vi "DrivePath.vi"(3 "Reinit":bool) -> (0 "Path Follower Error":errorcluster, 1 "Increment":bool)   [LabVIEW 2019]
doc: "A pure-pursuit path-following algorithm configured for a swerve drive. Feed-forward and feed-back controllers are combined to produce unitless drive commands. This VI is designed to integrated with the FRC 4265 Autonomous Path Planner. The Search Window can be specified in seconds - longer search windows are more robust to recovering from large deviations from the path but may cause the robot to \"jump\" ahead when following tight loops or turns. The Look-Ahead Time specifies the furthest ahead the pursuit point can be.\n\nParameters:\n1. acceptable distance error --> (in) [0,614.25]\n2. acceptable angle error --> (deg) [0,180]\n3. path follow timeout --> (ms) [0,15000] set to -1 for no timeout\n3. name of the autonomous path\n4. specifiy whether or not the robot can add a suffix to the selected path name {normal,robot_suffix}"
uses:
  sensors.vi
  dsinstructions.vi
  autoninfo.vi
panel:
  in  "Dist Kd":dbl
  in  "Turn Kd":dbl
  in  "Turn Ki":dbl
  in  "Turn Kp":dbl
  in  "Dist Ki":dbl
  in  "Dist Kp":dbl
  in  "file_name":string
  in  "timeout":dbl
  in  "acceptable angle error":dbl
  in  "acceptable distance error":dbl
  out "PID Strafe":cluster{"Goal Wheel Position":dbl, dbl}(graph)
  out "PID Heading":cluster{"Goal Wheel Position":dbl, dbl}(graph)
  out "Path and Robot Pose":cluster{dbl[], dbl[]}[](graph)
  in  "Plot":bool
  in  "Max Look-Ahead Time (s)":dbl=0.5
  in  "Search Window (s)":dbl=2.0
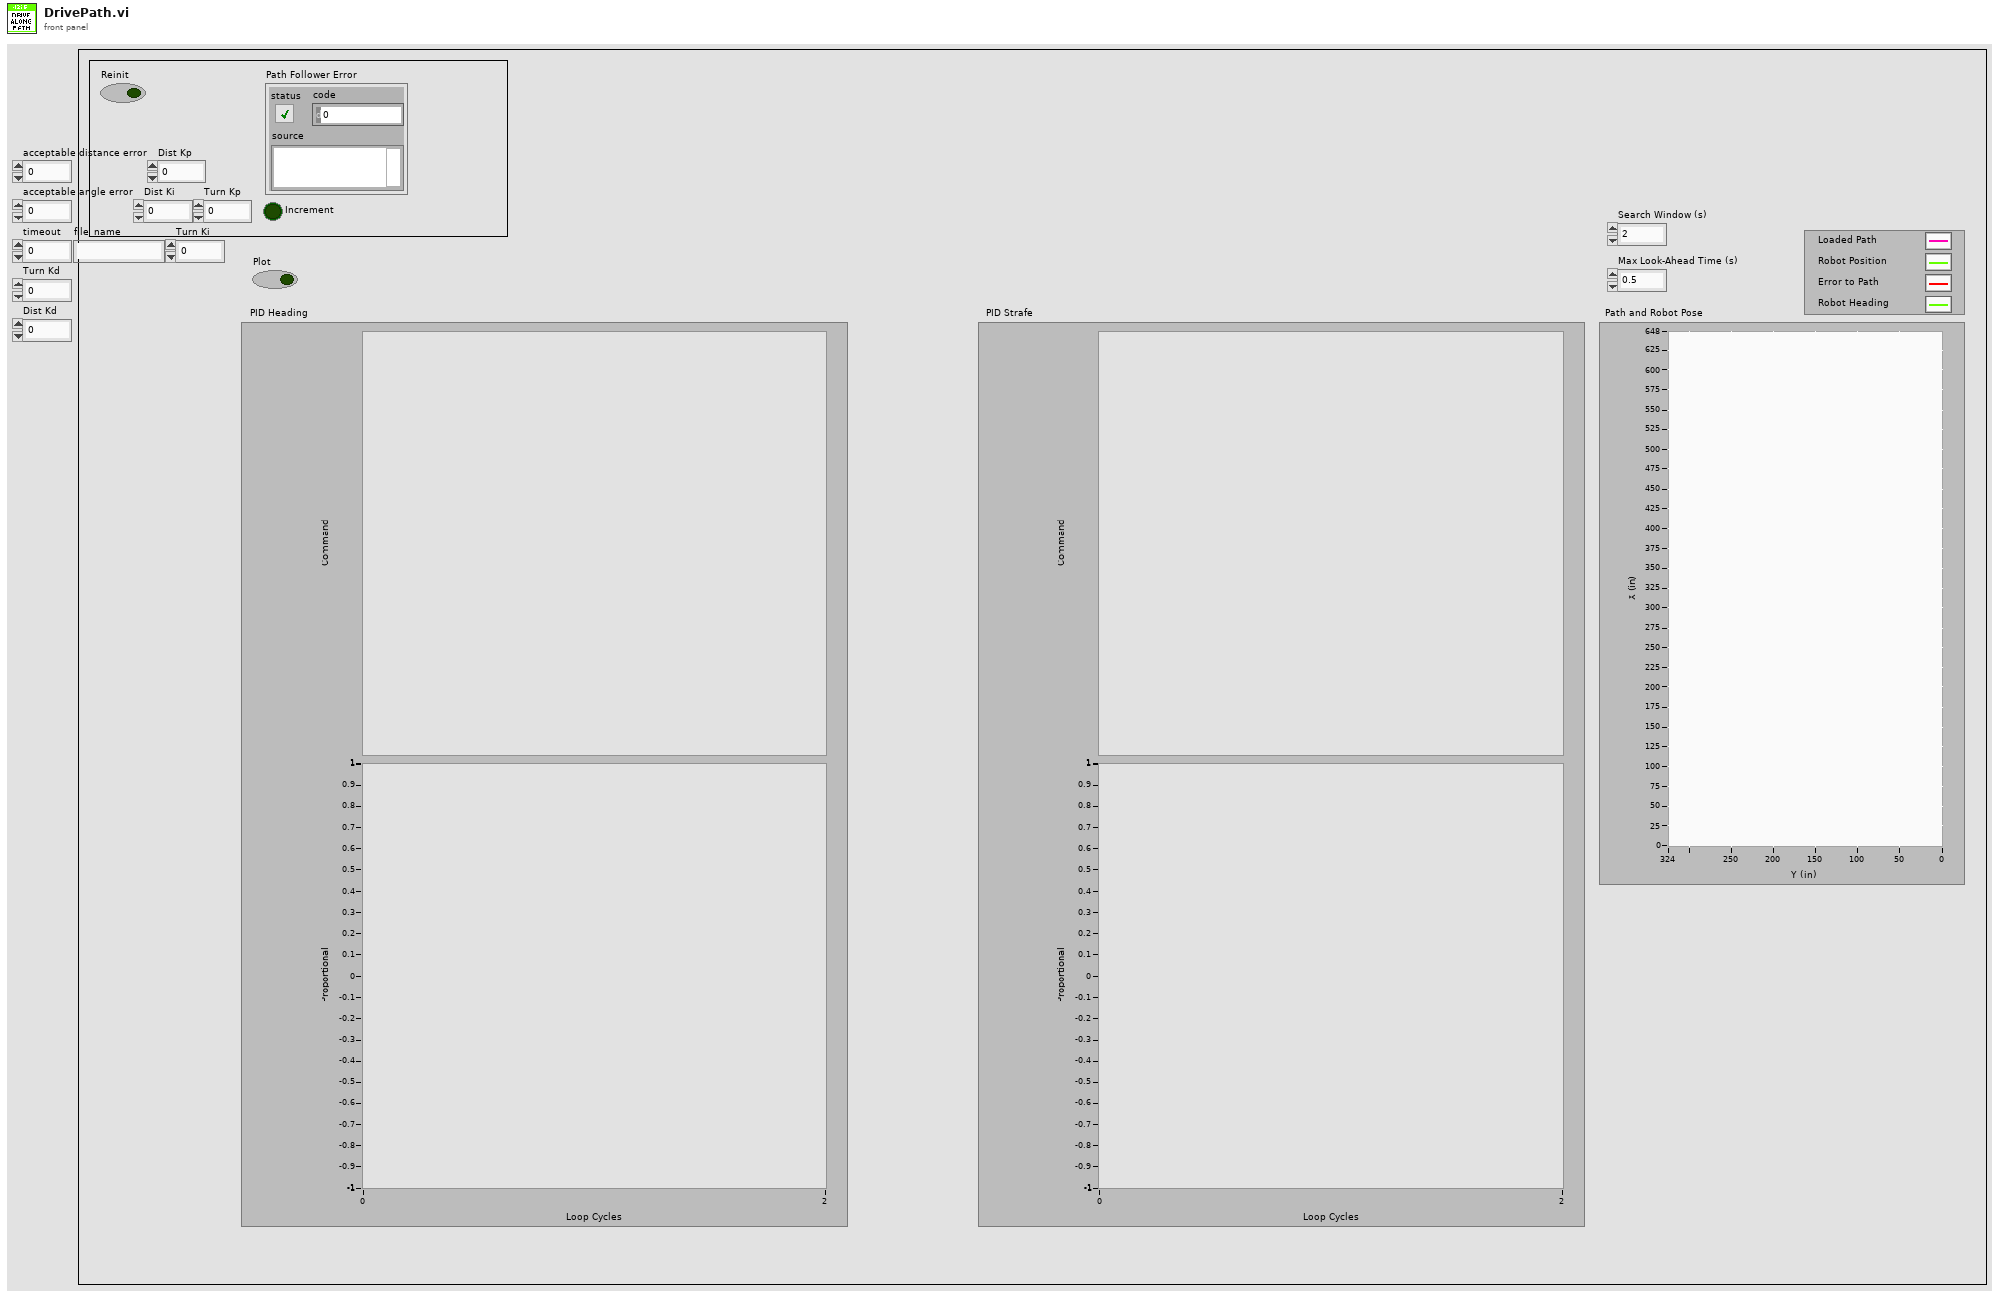
[diagram p1: front panel]
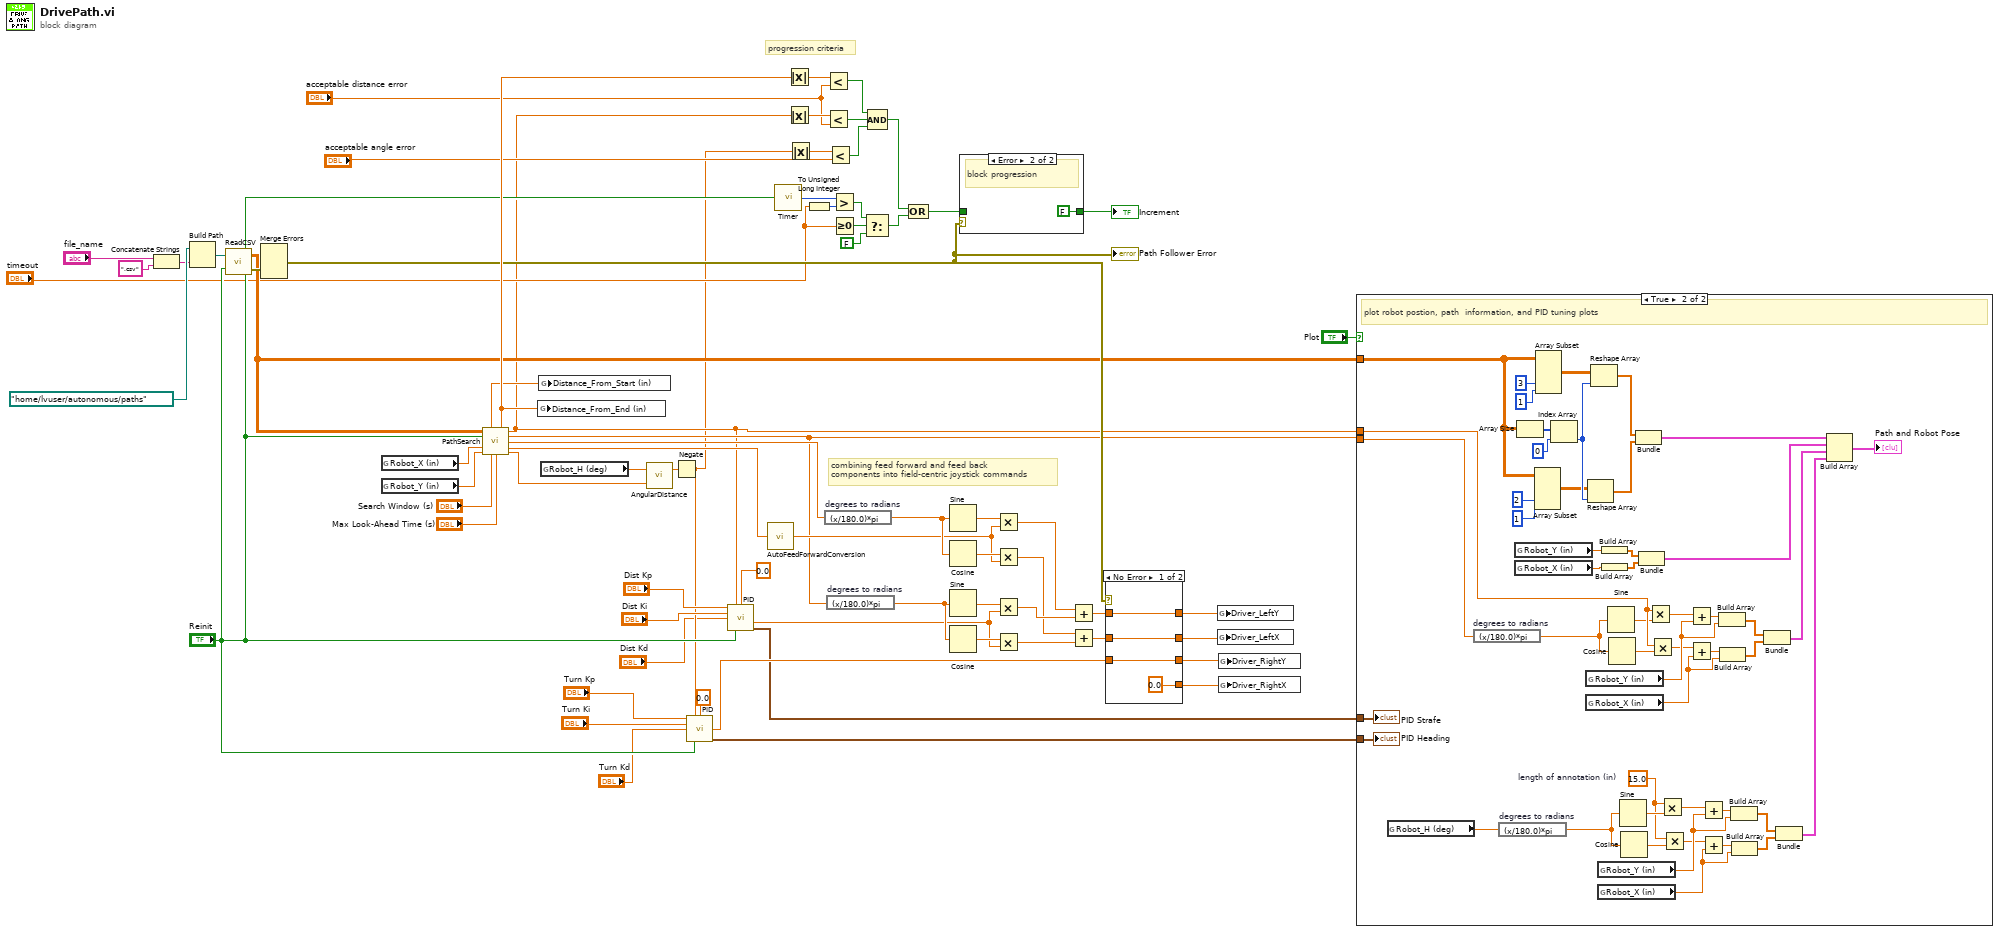
[diagram p0: block diagram]
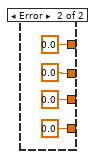
[diagram p4: hidden frame]
diagram:
  # "progression criteria"
  # "combining feed forward and feed back\ncomponents into field-centric joystick commands"
  n1 = Concatenate Strings("file_name", ".csv" ("string")) -> (w64:string)
  n2 = Build Path(base path=path "/home/lvuser/autonomous/paths" ("path"), name or relative path=w64) -> (appended path=w70:path)
  n3 = call "ReadCSV.vi"("Reinit"="Reinit", "File Path (.csv)"=w70) -> ("File Open Eror"=w45:errorcluster, "Data (index by row)"=w31:dbl[][])
  n4 = Merge Errors(w45) -> (w46:errorcluster)  [unwired: 4 in]
  "Path Follower Error" <- w46
  n5 = global read "sensors.vi" "Robot_X (in)"() -> (w69:dbl)
  n6 = global read "sensors.vi" "Robot_Y (in)"() -> (w68:dbl)
  n7 = call "PathSearch.vi"("Path"=w31, "Reint"="Reinit", "Robot X (in)"=w69, "Robot Y (in)"=w68, "Search Window (s)"="Search Window (s)", "Look-Ahead Time (s)"="Max Look-Ahead Time (s)") -> ("Distance from Start (in)"=w57:dbl, "Distance from End (in)"=w58:dbl, "Feed Back Distance Error (in)"=w5:dbl, "Feed Back Pointing Angle (deg)"=w22:dbl, "Feed Forward Pointing Angle (deg)"=w27:dbl, "Feed Forward Velocity (in/s)"=w59:dbl, "Robot Heading Goal (deg)"=w47:dbl)  [unwired: 3 in]
  n8 = global write "autoninfo.vi" "Distance_From_End (in)"(w58) -> ()
  n9 = global write "autoninfo.vi" "Distance_From_Start (in)"(w57) -> ()
  n10 = global read "sensors.vi" "Robot_H (deg)"() -> (w42:dbl)
  n11 = call "AngularDistance.vi"("Goal Angle (deg) [0,360]"=w47, "Current Angle (deg) [-Inf,+Inf]"=w42) -> ("Signed Angular Distance (deg) [-180,+180]"=w40:dbl)  [unwired: 1 out]
  n12 = Negate(x=w40) -> (-x=w3:dbl)
  n13 = call "PID.vi"("Kp"="Turn Kp", "Process Variable"=w3, "Goal"=0.0, "Ki"="Turn Ki", "Kd"="Turn Kd", "Reinit"="Reinit") -> ("Command"=w44:dbl, "PID Tracking"=w39:cluster{"Goal Wheel Position":dbl, dbl})  [unwired: 7 in, 1 out]
  n14 = call "PID.vi"("Kp"="Dist Kp", "Process Variable"=w5, "Goal"=0.0, "Ki"="Dist Ki", "Kd"="Dist Kd", "Reinit"="Reinit") -> ("Command"=w21:dbl, "PID Tracking"=w43:cluster{"Goal Wheel Position":dbl, dbl})  [unwired: 7 in, 1 out]
  n15 = call "AutoFeedForwardConversion.vi"("Target Velocity (in/s)"=w59) -> ("Equivalent Joystick Command (ul)"=w26:dbl)
  n16 = call "Timer.vi"("Reset Timer"="Reinit") -> ("Time (ms)"=w48:u32)
  n17 = Absolute Value(x=w58) -> (abs(x)=w49:dbl)
  n18 = Absolute Value(x=w5) -> (abs(x)=w50:dbl)
  n19 = Absolute Value(x=w3) -> (abs(x)=w56:dbl)
  n20 = To Unsigned Long Integer(number="timeout") -> (unsigned 32bit integer=w54:u32)
  n21 = expression code="(x/180.0)*pi" "degrees to radians"(w27) -> (w62:dbl)
  n22 = Less?(x=w49, y="acceptable distance error") -> (x < y?=w34:bool)
  n23 = Less?(x=w50, y="acceptable distance error") -> (x < y?=w35:bool)
  n24 = Less?(x=w56, y="acceptable angle error") -> (x < y?=w36:bool)
  n25 = expression code="(x/180.0)*pi" "degrees to radians"(w22) -> (w25:dbl)
  n26 = Greater?(x=w48, y=w54) -> (0:w52:bool)
  n27 = Greater Or Equal To 0?(x="timeout") -> (x >= 0?=w53:bool)
  n28 = Select(t=w52, s=w53, f=FALSE) -> (s? t:f=w32:bool)
  n29 = Compound Arithmetic op=AND(w34, w35, w36) -> (w33:bool)
  n30 = Compound Arithmetic op=OR(w33, w32) -> (w55:bool)
  n31 = Sine(x=w62) -> (sin(x)=w61:dbl)
  n32 = Cosine(x=w62) -> (cos(x)=w60:dbl)
  n33 = Sine(x=w25) -> (sin(x)=w24:dbl)
  n34 = Cosine(x=w25) -> (cos(x)=w23:dbl)
  n35 = case shown="Error" w46 {
    tunnel: [w72 FALSE] -> w65
    tunnel: w55 -> [w72 _]
    frame No Error {
      # "allow progression"
    }
    frame Error {
      # "block progression"
    }
  }
  "Increment" <- w65
  n36 = Multiply(x=w61, y=w26) -> (x*y=w20:dbl)
  n37 = Multiply(x=w60, y=w26) -> (x*y=w18:dbl)
  n38 = Multiply(x=w24, y=w21) -> (x*y=w19:dbl)
  n39 = Multiply(x=w23, y=w21) -> (x*y=w17:dbl)
  n40 = Add(x=w20, y=w19) -> (x+y=w16:dbl)
  n41 = Add(x=w18, y=w17) -> (x+y=w15:dbl)
  n42 = case shown="No Error" w46 {
    tunnel: [w74 0.0] -> w38
    tunnel: [w77 0.0 ("upper limit")] -> w63
    tunnel: [w75 0.0] -> w37
    tunnel: w44 -> [w77 _]
    tunnel: [0.0 0.0] -> w41
    tunnel: w16 -> [w75 _]
    tunnel: w15 -> [w74 _]
    frame No Error {
    }
    frame Error {
    }
  }
  n43 = global write "dsinstructions.vi" "Driver_LeftY"(w37) -> ()
  n44 = global write "dsinstructions.vi" "Driver_LeftX"(w38) -> ()
  n45 = global write "dsinstructions.vi" "Driver_RightY"(w63) -> ()
  n46 = global write "dsinstructions.vi" "Driver_RightX"(w41) -> ()
  n47 = case shown="True" "Plot" {
    tunnel: w22 -> [_ w125]
    tunnel: w43 -> [_ w124]
    tunnel: w39 -> [_ w123]
    tunnel: w5 -> [_ w122]
    tunnel: w31 -> [_ w121]
    frame False {
    }
    frame True {
      w86 = 15.0  # length of annotation (in)
      # "plot robot postion, path  information, and PID tuning plots"
      n48 = global read "sensors.vi" "Robot_H (deg)"() -> (w126:dbl)
      n49 = expression code="(x/180.0)*pi" "degrees to radians"(w125) -> (w98:dbl)
      n50 = expression code="(x/180.0)*pi" "degrees to radians"(w126) -> (w87:dbl)
      n51 = global read "sensors.vi" "Robot_Y (in)"() -> (w130:dbl)
      n52 = global read "sensors.vi" "Robot_X (in)"() -> (w129:dbl)
      n53 = Array Size(array=w121) -> (size(s)=w117:i32[])
      n54 = Array Subset(array=w121, index (col)=2 ("index"), length (col)=1 ("length")) -> (w115:dbl[][])  [unwired: 2 in]
      n55 = Array Subset(array=w121, index (col)=3 ("index"), length (col)=1 ("length")) -> (w116:dbl[][])  [unwired: 2 in]
      n56 = Index Array(array=w117, index=0) -> (element=w118:i32)
      n57 = global read "sensors.vi" "Robot_Y (in)"() -> (w108:dbl)
      n58 = global read "sensors.vi" "Robot_X (in)"() -> (w107:dbl)
      n59 = Reshape Array(w115, w118) -> (w83:dbl[])
      n60 = Reshape Array(w116, w118) -> (w84:dbl[])
      n61 = global read "sensors.vi" "Robot_Y (in)"() -> (w97:dbl)
      n62 = global read "sensors.vi" "Robot_X (in)"() -> (w96:dbl)
      n63 = Build Array(w130) -> (w127:dbl[])
      n64 = Build Array(w129) -> (w128:dbl[])
      n65 = Sine(x=w98) -> (sin(x)=w99:dbl)
      n66 = Cosine(x=w98) -> (cos(x)=w100:dbl)
      n67 = Sine(x=w87) -> (sin(x)=w88:dbl)
      n68 = Cosine(x=w87) -> (cos(x)=w89:dbl)
      n69 = Bundle(w84, w83) -> (w120:cluster{dbl[], dbl[]})  [unwired: 1 in]
      n70 = Bundle(w127, w128) -> (w109:cluster{dbl[], dbl[]})  [unwired: 1 in]
      n71 = Multiply(x=w122, y=w99) -> (x*y=w101:dbl)
      n72 = Multiply(x=w122, y=w100) -> (x*y=w102:dbl)
      n73 = Multiply(x=w86, y=w88) -> (x*y=w90:dbl)
      n74 = Multiply(x=w86, y=w89) -> (x*y=w91:dbl)
      n75 = Add(x=w101, y=w108) -> (x+y=w103:dbl)
      n76 = Add(x=w102, y=w107) -> (x+y=w104:dbl)
      n77 = Add(x=w90, y=w97) -> (x+y=w92:dbl)
      n78 = Add(x=w91, y=w96) -> (x+y=w93:dbl)
      n79 = Build Array(w103, w108) -> (w105:dbl[])
      n80 = Build Array(w104, w107) -> (w106:dbl[])
      n81 = Build Array(w92, w97) -> (w94:dbl[])
      n82 = Build Array(w93, w96) -> (w95:dbl[])
      n83 = Bundle(w105, w106) -> (w85:cluster{dbl[], dbl[]})  [unwired: 1 in]
      n84 = Bundle(w94, w95) -> (w82:cluster{dbl[], dbl[]})  [unwired: 1 in]
      n85 = Build Array(w120, w109, w85, w82) -> (→"Path and Robot Pose":cluster{dbl[], dbl[]}[])
      "PID Strafe" <- w124
      "PID Heading" <- w123
    }
  }
